vi "AzCam.vi"(0 "Command":string) -> (1 "Error":bool, 2 "Reply":string)   [LabVIEW 2014]
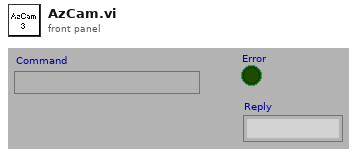
[diagram p1: front panel]
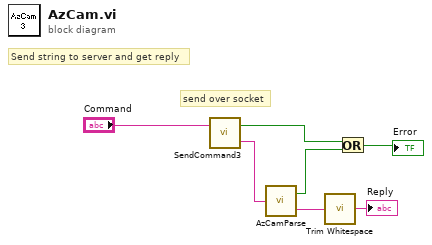
[diagram p0: block diagram]
diagram:
  # "send over socket"
  # "Send string to server and get reply"
  n1 = call "SendCommand3.vi"("command"="Command") -> ("reply"=w7:string, "Error"=w1:bool)  [unwired: 1 in]
  n2 = call "AzCamParse.vi"("InputString"=w7) -> ("Error"=w3:bool, "Reply"=w4:string)
  n3 = call <vilib>:"Trim Whitespace.vi"("string"=w4) -> ("trimmed string"=→"Reply":string)  [unwired: 1 in]
  n4 = Or(x=w1, y=w3) -> (x .or. y?=→"Error":bool)
